vi "DisplayLogic_DrawScore.vi"(0 "Player":u8, 1 "ActivePixel":cluster{"h_pixel":i16, "v_pixel":i16}, 4 "ScorePosition":T1) -> (16 "PixelData":bool[](array[boolean]))   [LabVIEW 2018]
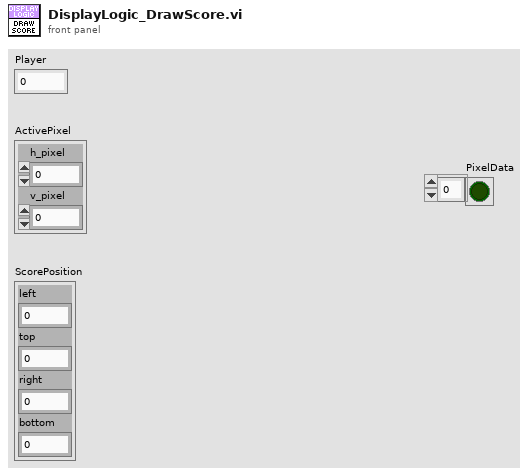
[diagram p1: front panel]
types:
  T1 = cluster{"left":i16, "top":i16, "right":i16, "bottom":i16}
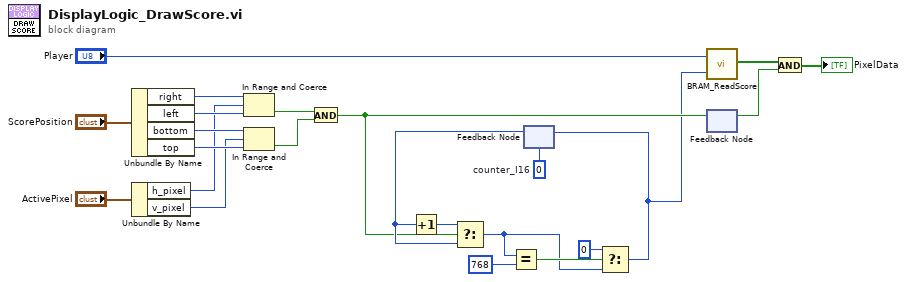
[diagram p0: block diagram]
diagram:
  w9 = i16 0  # counter_I16
  n1 = Unbundle By Name("ScorePosition") -> ("right"=w20:i16, "left"=w19:i16, "bottom"=w18:i16, "top"=w13:i16)
  n2 = Unbundle By Name("ActivePixel") -> ("h_pixel"=w11:i16, "v_pixel"=w12:i16)
  n3 = In Range and Coerce(upper limit=w20, x=w11, lower limit=w19) -> (In Range?=w17:bool)  [unwired: 1 out]
  n4 = In Range and Coerce(upper limit=w18, x=w12, lower limit=w13) -> (In Range?=w16:bool)  [unwired: 1 out]
  n5 = And(x=w17, y=w16) -> (x .and. y?=w3:bool)
  n6 = feedback #1(w9) -> (w4:i16)
  n7 = Increment(x=w4) -> (x+1=w7:i16)
  n8 = Select(t=w7, s=w3, f=w4) -> (s? t:f=w6:i16)
  n9 = Equal?(x=w6, y=i16 768) -> (x = y?=w8:bool)
  n10 = Select(t=i16 0 ("f"), s=w8, f=w6) -> (s? t:f=w2:i16)
  n11 = feedback-in #1(w2) -> ()
  n12 = call "BRAM_ReadScore.vi"("Player"="Player", "Address"=w2) -> ("PixelData"=w23:bool[])  [unwired: 17 in]
  n13 = feedback #2() -> (w1:bool)  [unwired: 1 in]
  n14 = feedback-in #2(w3) -> ()
  n15 = And(x=w23, y=w1) -> (x .and. y?=→"PixelData":bool[])
